vi "WriteFile.vi"(8 "error in (no error)":errorcluster, 10 "data":i32[](array[numeric]), 11 "File in":refnum<class "File.lvclass">) -> (0 "error out":errorcluster, 3 "File out":refnum<class "File.lvclass">)   [LabVIEW 2021, in "File.lvclass"]
uses:
  File.lvclass
  File.lvclass/File.ctl
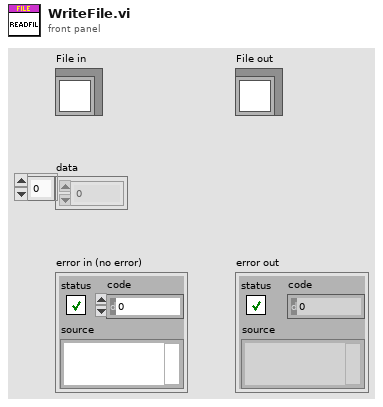
[diagram p1: front panel]
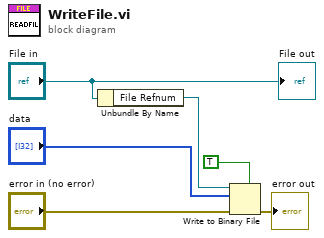
[diagram p0: block diagram]
diagram:
  n1 = Unbundle By Name("File in") -> ("File Refnum"=w3:refnum<file>)
  n2 = Write to Binary File(file (use dialog)=w3, data="data", error in="error in (no error)", 5:TRUE ("prepend array or string size? (T)")) -> (error out=→"error out":errorcluster)  [unwired: 2 in, 2 out]
  "File out" <- "File in"
